vi "3D-SaveLaserParams.vi"(8 "Motion Cal Collect":string[][](table)=[["", "", ""], ["", "", ""]], 9 "Motion  Data Collect":string[][](table)=[["", "", ""], ["", "", ""]], 10 "名称或相对路径":string, 11 "路径":path) -> ()   [LabVIEW 2017]
uses:
  <vilib>/Utility/file.llb/Write To Spreadsheet File (string).vi
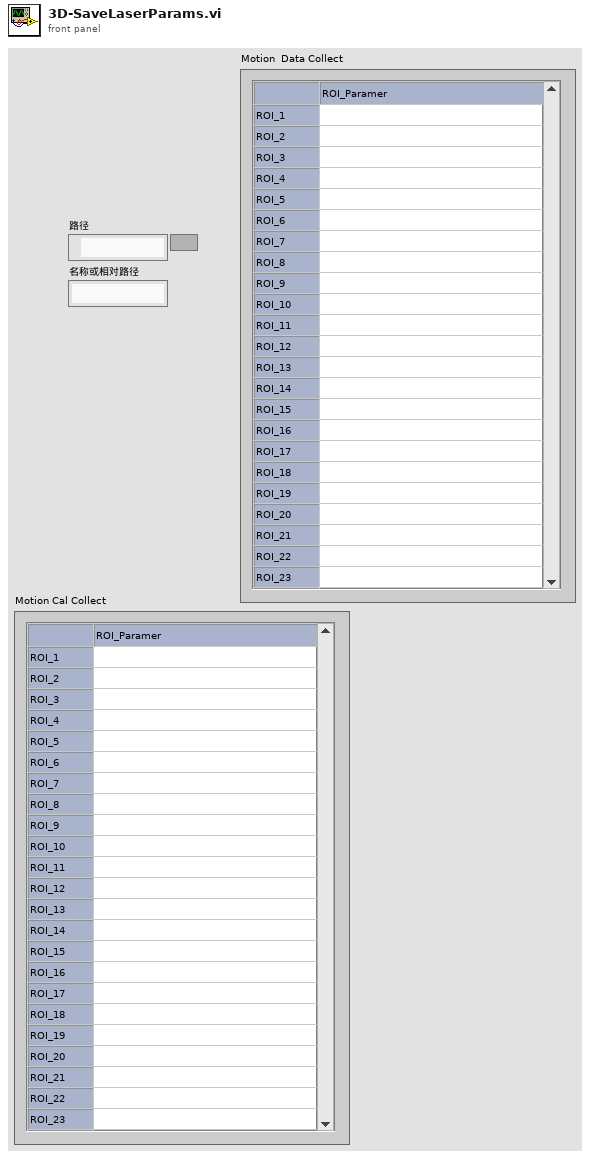
[diagram p1: front panel]
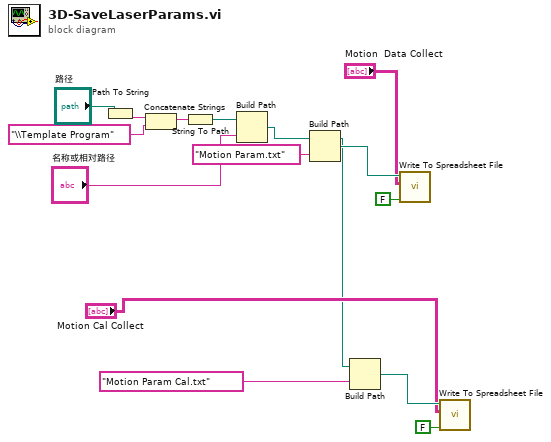
[diagram p0: block diagram]
diagram:
  n1 = Path To String(path="路径") -> (string=w15:string)
  n2 = Concatenate Strings(w15, "\\Template Program" ("字符串")) -> (w14:string)
  n3 = String To Path(string=w14) -> (path=w12:path)
  n4 = Build Path(base path=w12, name or relative path="名称或相对路径") -> (appended path=w2:path)
  n5 = Build Path(base path=w2, name or relative path="Motion Param.txt" ("名称或相对路径")) -> (appended path=w7:path)
  n6 = Build Path(base path=w2, name or relative path="Motion Param Cal.txt" ("名称或相对路径")) -> (appended path=w5:path)
  n7 = call-poly <vilib>:"Write To Spreadsheet File.vi"("append to file? (new file:F)"=FALSE, "2D data"="Motion  Data Collect", "file path (dialog if empty)"=w7) -> ()  [unwired: 5 in, 1 out]
  n8 = call-poly <vilib>:"Write To Spreadsheet File.vi"("append to file? (new file:F)"=FALSE, "2D data"="Motion Cal Collect", "file path (dialog if empty)"=w5) -> ()  [unwired: 5 in, 1 out]
